vi "Teardown.vi"(8 "error in (no error)":errorcluster, 11 "LUnit Tear Down Error In":refnum<class "LUnit Tear Down Error.lvclass">) -> (0 "error out":errorcluster, 3 "LUnit Tear Down Error Out":refnum<class "LUnit Tear Down Error.lvclass">)   [LabVIEW 2020, in "LUnit Tear Down Error.lvclass"]
uses:
  LUnit Tear Down Error.lvclass
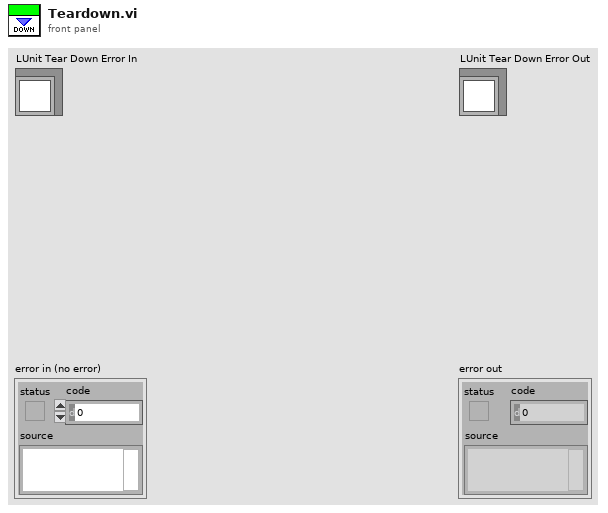
[diagram p1: front panel]
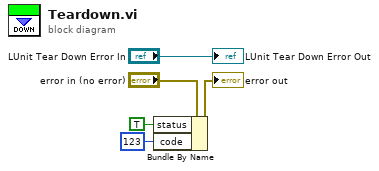
[diagram p0: block diagram]
diagram:
  n1 = Bundle By Name(cluster="error in (no error)", "status"=TRUE, "code"=123) -> (→"error out":errorcluster)
  "LUnit Tear Down Error Out" <- "LUnit Tear Down Error In"
